vi "Make In, Out Channels.vi"(0 "AI Configuration In":T2(array[cluster])=[{"AI.Coupling"=10050, "AI.Max"=10.0, "AI.Min"=-10.0, "Input physical channels"="PXI1Slot2/ai0:1"}, {"AI.Coupling"=10050, "AI.Max"=10.0, "AI.Min"=-10.0, "Input physical channels"="PXI1Slot3/ai0:3"}, {"AI.Coupling"=10050, "AI.Max"=10.0, "AI.Min"=-10.0, "Input physical channels"=""}] {"AI.Coupling" items=["AC"=10045, "DC"=10050, "GND"=10066]}, 1 "AI Buffer Size (s) In":i32=10, 5 "AO Configuration Out":T1(array[cluster])=[{"Output physical channels"="PXI1Slot2/ao0", "AO. Max"=0.1, "AO.Min"=-0.1}, {"Output physical channels"="", "AO. Max"=0.1, "AO.Min"=-0.1}], 7 "Num. of Cards":i32=2, 9 "OSC Configuration In":T3(array[cluster])=[[{"Signal Type"=enum."Sine Wave", "DC"=0.0, "Amplitude"=0.001, "frequency"=2.0, "Phase"=0.0}, {"Signal Type"=enum."Sine Wave", "DC"=0.0, "Amplitude"=0.0, "frequency"=2.0, "Phase"=0.0}, {"Signal Type"=enum."Sine Wave", "DC"=0.0, "Amplitude"=0.0, "frequency"=20.0, "Phase"=0.0}], [{"Signal Type"=enum."Sine Wave", "DC"=0.0, "Amplitude"=0.0, "frequency"=2.0, "Phase"=0.0}, {"Signal Type"=enum."Sine Wave", "DC"=0.0, "Amplitude"=0.0, "frequency"=2.0, "Phase"=0.0}, {"Signal Type"=enum."Sine Wave", "DC"=0.0, "Amplitude"=0.0, "frequency"=20.0, "Phase"=0.0}]] {"frequency" step=0.001 format="%.3p"; "Amplitude" format="%0.2p"; "DC" min=-0.99 max=0.99 format="%.2p"}, 11 "AI Block Size In":i32=5000) -> (4 "AI Task Out":refnum<k21>[](array[refnum]), 6 "AO Task Out":refnum<k21>[](array[refnum]), 8 "Phase Log Out":dbl[](array[numeric])=[0.9999999999893834, 0.9999999999893834], 10 "AI Rate Out":dbl=10000.0 format="%.2f", 15 "Sampling Information Out":cluster{"Fs":dbl, "#s":dbl}[](array[cluster])=[{"Fs"=10000.0, "#s"=5000.0}, {"Fs"=10000.0, "#s"=5000.0}])   [LabVIEW 2013, in "Lock-In Variable Channels_2.lvclass"]
uses:
  Lock-In Variable Channels_2.lvclass
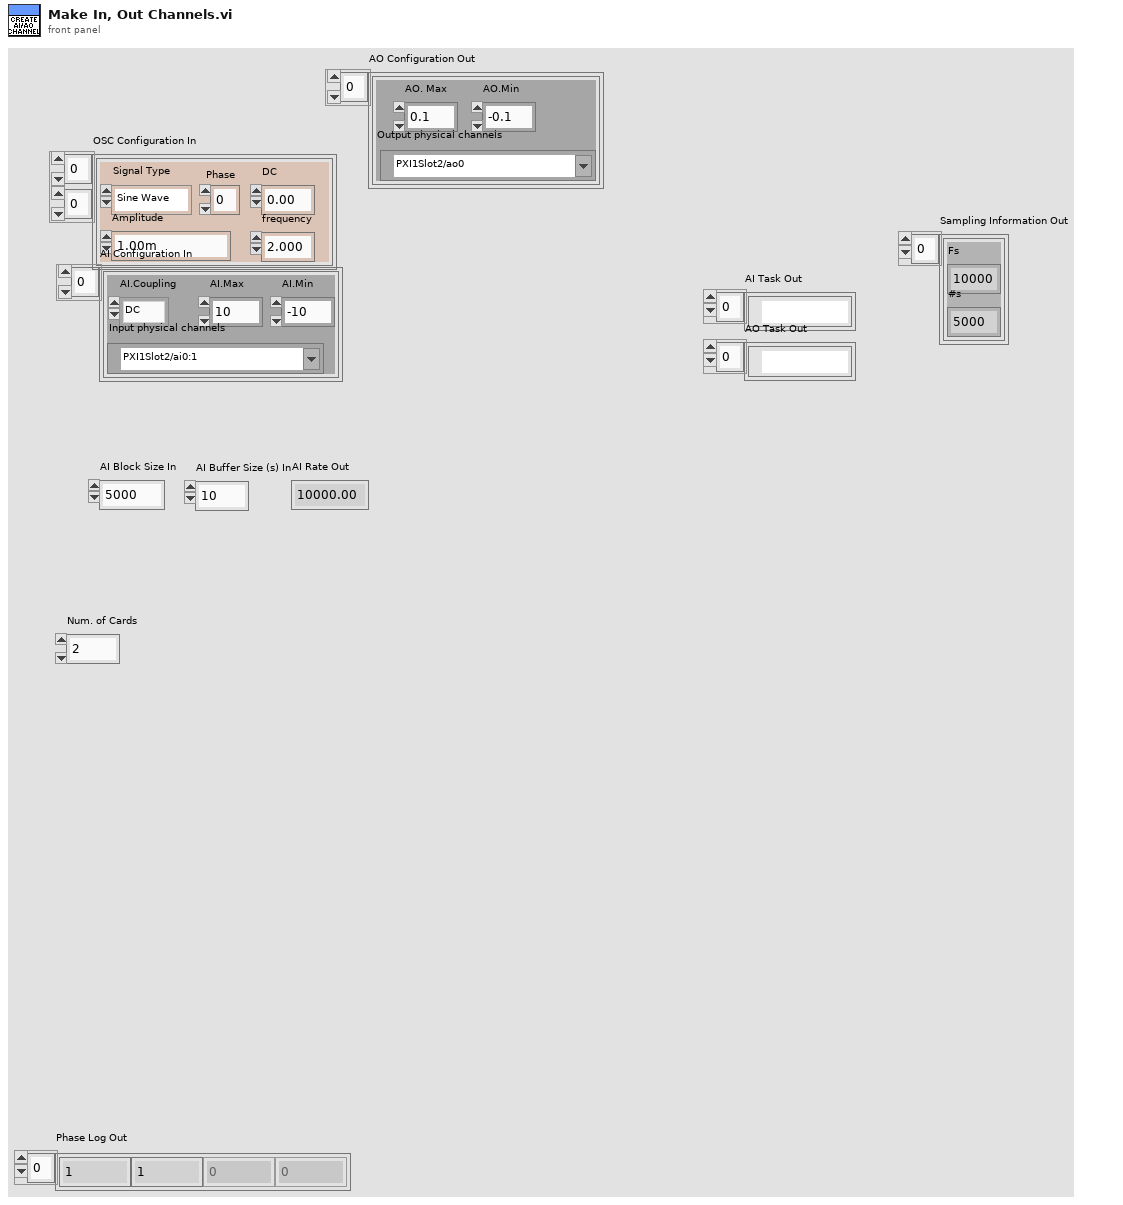
[diagram p1: front panel]
types:
  T1 = cluster{"Output physical channels":tag, "AO. Max":dbl, "AO.Min":dbl}[]
  T2 = cluster{"AI.Coupling":i32, "AI.Max":dbl, "AI.Min":dbl, "Input physical channels":tag}[]
  T3 = cluster{"Signal Type":enum16{"Sine Wave", "Triangle Wave", "Square Wave", "Sawtooth Wave"}, "DC":dbl, "Amplitude":dbl, "frequency":dbl, "Phase":dbl}[][]
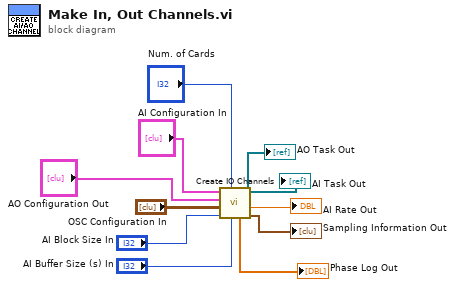
[diagram p0: block diagram]
diagram:
  n1 = call "Create IO Channels.vi"("AI Buffer Size (s)"="AI Buffer Size (s) In", "Num. of Cards"="Num. of Cards", "AI Block Size"="AI Block Size In", "OSC Configuration"="OSC Configuration In", "AO Configuration"="AO Configuration Out", "AI Configuration"="AI Configuration In") -> ("Sampling information"=→"Sampling Information Out":cluster{"Fs":dbl, "#s":dbl}[], "AI Rate"=→"AI Rate Out":dbl, "AO Task"=→"AO Task Out":refnum<k21>[], "AI task"=→"AI Task Out":refnum<k21>[], "phase log"=→"Phase Log Out":dbl[])  [unwired: 1 in]
